vi "InitializeAnalogOutputforPADwithRamp.vi"(0 "AOTF":u16(ring) items=["None", "Laser 1", "Laser 2", "Laser 1 + 2", "Laser 3", "Laser 1 + 3", "Laser 2 + 3", "Laser 1+2+3", "Laser 1+2+3+4", "Laser 2+3+4"]) -> ()   [LabVIEW 2009]
uses:
  AnalogTrace.ctt
  TimingInfo.ctt
  <vilib>/Waveform/WDTOps.llb/WDT Append Waveforms DBL.vi
panel:
  in  "signal out":waveform(dbl)={"t0"=timestamp(0 s since 1904-01-01), "dt"=0.0, "Y"=[]}
  in  "Trace":T1
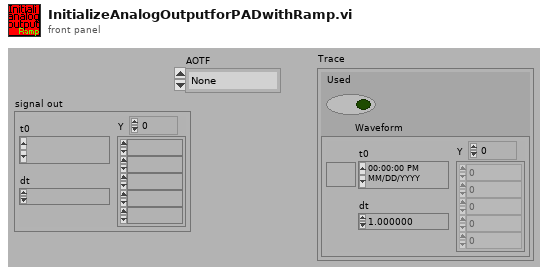
[diagram p1: front panel]
types:
  T1 = typedef "AnalogTrace.ctt" = cluster{"Used":bool, "Waveform":waveform(dbl)}
  T2 = cluster{"used":bool, "steps":u16, "start (V)":dbl, "stop (V)":dbl, "periode (s)":dbl, "manual":dbl[][]}
  T3 = typedef "TimingInfo.ctt" = cluster{"Fs":dbl, "#s":dbl}
  T4 = typedef "FIFOSettings.ctt" = cluster{"Measurement":cluster{"Binning (ms)":sgl, "External Trigger Condition":u16, "Stop Condition:":u16, "Stop Count":dbl, "Buffer Size (Photons)":u32, "No of Channels":u16, "Ext Latch Delay":i16}, "ADC":cluster{"Binning (HH)":i16, "Dither Range":i16, "Count Increment":i16, "Mode":u16}, "SYNC":cluster{"SYNC ZC Level (mV)":sgl, "SYNC Freq Divider":u16, "SYNC Holdoff (ps)":sgl, "SYNC Threshold (mV)":sgl}, "TAC":cluster{"TAC Range (ns)":sgl, "TAC Gain":i16, "TAC Offset (%)":sgl, "TAC Limit Low (%)":sgl, "TAC Limit High (%)":sgl}, "Ch 2":cluster{"Ch2 ZC Level (mV)":sgl, "Ch2 Holdoff (ps)":sgl, "Ch2 Threshold (mV)":sgl}, "Ch 3":cluster{"Ch3 ZC Level (mV)":sgl, "Ch3 Holdoff (ps)":sgl, "Ch3 Threshold (mV)":sgl}, "Ch 4":cluster{"Ch4 ZC Level (mV)":sgl, "Ch4 Holdoff (ps)":sgl, "Ch4 Threshold (mV)":sgl}, "Ch1":cluster{"Ch1 ZC Level (mV)":sgl, "Ch1 Holdoff (ps)":sgl, "Ch1 Threshold (mV)":sgl}}
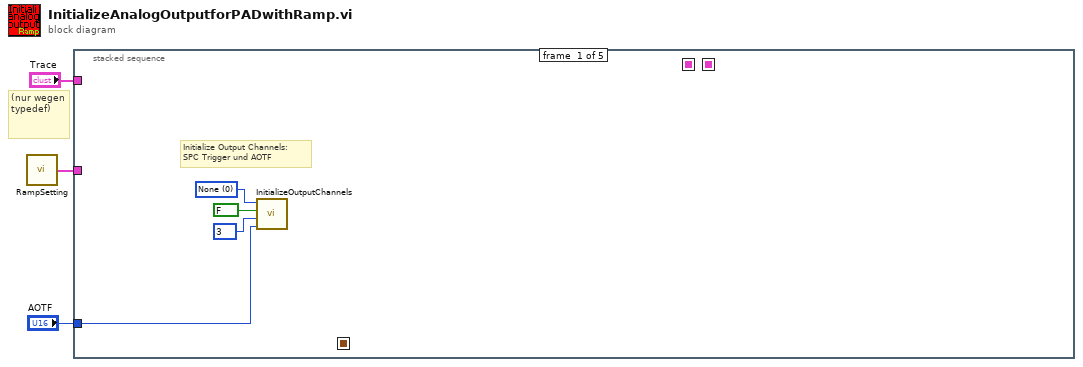
[diagram p0: block diagram]
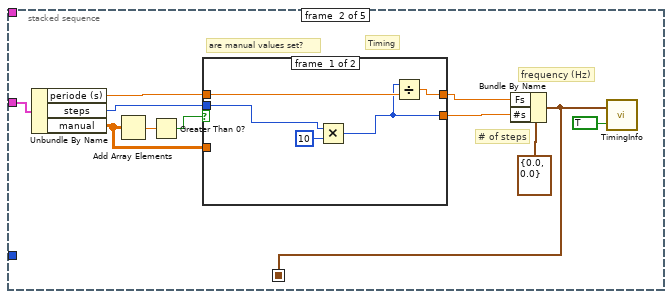
[diagram p2: hidden frame]
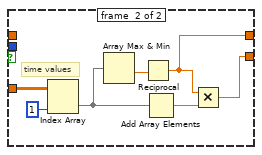
[diagram p3: hidden frame]
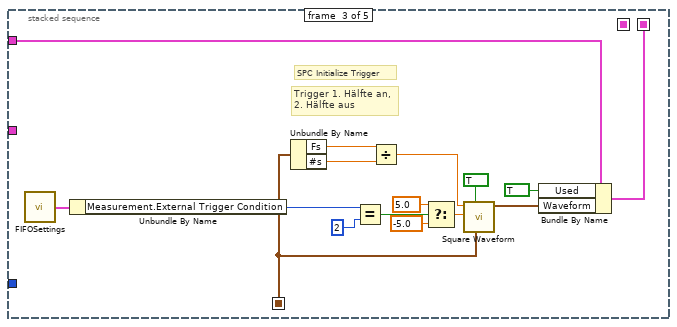
[diagram p4: hidden frame]
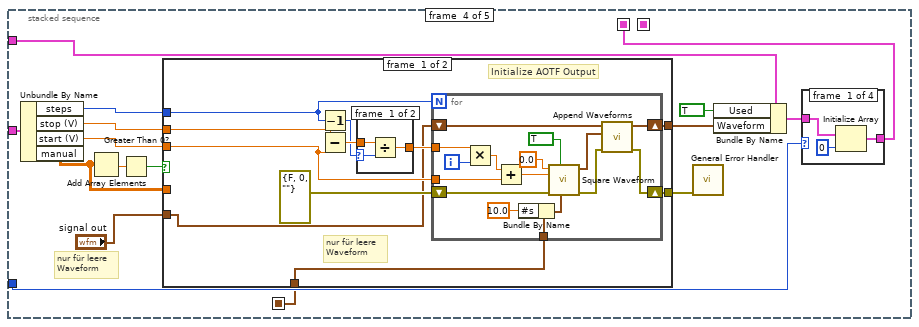
[diagram p5: hidden frame]
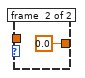
[diagram p6: hidden frame]
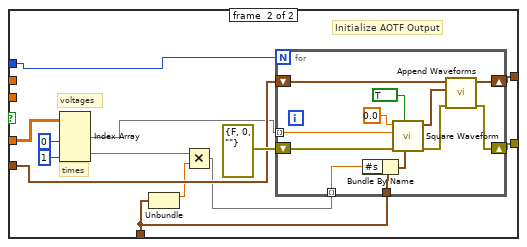
[diagram p7: hidden frame]
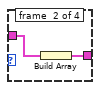
[diagram p8: hidden frame]
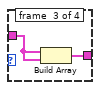
[diagram p9: hidden frame]
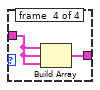
[diagram p10: hidden frame]
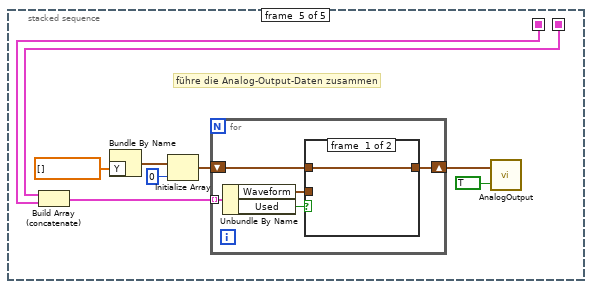
[diagram p11: hidden frame]
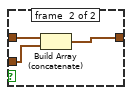
[diagram p12: hidden frame]
diagram:
  # "(nur wegen typedef)"
  n1 = call "RampSetting.vi"() -> ("RampSetting (out)"=w2:T2)  [unwired: 2 in]
  n2 = stacked-sequence {
    seq-local: [_ w15 _ _ _] -> [_ _ w35 w54 _]
    seq-local: [_ _ w34 _ _] -> [_ _ _ _ w129]
    seq-local: [_ _ _ w55 _] -> [_ _ _ _ w128]
    tunnel: "AOTF" -> [w4 _ _ w57 _]
    tunnel: w2 -> [_ w16 _ w56 _]
    tunnel: "Trace" -> [_ _ w33 w51 _]
    frame #0 {
      w7 = u16 0 items=["None", "Trace", "Retrace", "All"] ("EOM")
      w6 = u16 3 items=["x", "y", "z", ""] ("1st Axis")
      # "Initialize Output Channels:\nSPC Trigger und AOTF"
      n3 = call "InitializeOutputChannels.vi"("AOTF"=w4, "1st Axis"=w6, "Retrace"=FALSE, "EOM"=w7) -> ()
    }
    frame #1 {
      # "# of steps"
      # "frequency (Hz)"
      # "are manual values set?"
      # "Timing"
      n4 = Unbundle By Name(w16) -> ("periode (s)"=w13:dbl, "steps"=w12:u16, "manual"=w10:dbl[][])
      n5 = Add Array Elements(numeric array=w10) -> (sum=w14:dbl)
      n6 = Greater Than 0?(x=w14) -> (x > 0?=w11:bool)
      n7 = case shown="True" w11 {
        tunnel: [w19 w25] -> w8
        tunnel: w13 -> [w21 _]
        tunnel: [w20 w24] -> w9
        tunnel: w12 -> [w22 _]
        tunnel: w10 -> [_ w29]
        frame #0 {
          n8 = Multiply(x=w22, y=u16 10) -> (x*y=w20:u16)
          n9 = Divide(x=w20, y=w21) -> (x/y=w19:dbl)
        }
        frame #1 {
          # "time values"
          n10 = Index Array(array=w29, index (col)=1 ("disabled index (col)")) -> (element=w27:dbl[])  [unwired: 1 in]
          n11 = Array Max & Min(array=w27) -> (min value=w28:dbl)  [unwired: 3 out]
          n12 = Reciprocal(x=w28) -> (1/x=w25:dbl)
          n13 = Add Array Elements(numeric array=w27) -> (sum=w26:dbl)
          n14 = Multiply(x=w25, y=w26) -> (x*y=w24:dbl)
        }
      }
      n15 = Bundle By Name(cluster=T3 {"Fs"=0.0, "#s"=0.0} ("Timing Info"), "Fs"=w8, "#s"=w9) -> (w15:T3)
      n16 = call "TimingInfo.vi"("Get/Set"=TRUE, "Timing Info (input)"=w15) -> ()  [unwired: 1 out]
    }
    frame #2 {
      # "Trigger 1. Hälfte an, 2. Hälfte aus"
      # "SPC Initialize Trigger"
      n17 = call "FIFOSettings.vi"() -> ("FIFO Settings(out)"=w36:T4)  [unwired: 2 in]
      n18 = Unbundle By Name(w36) -> ("Measurement.External Trigger Condition"=w37:u16)
      n19 = Unbundle By Name(w35) -> ("Fs"=w46:dbl, "#s"=w32:dbl)
      n20 = Equal?(x=w37, y=u16 2) -> (x = y?=w41:bool)
      n21 = Divide(x=w46, y=w32) -> (x/y=w31:dbl)
      n22 = Select(t=5.0, s=w41, f=-5.0) -> (s? t:f=w45:dbl)
      n23 = call "Square Waveform.vi"("sampling info"=w35, "reset signal"=TRUE, "amplitude"=w45, "frequency"=w31) -> ("signal out"=w44:waveform(dbl))  [unwired: 6 in, 1 out]
      n24 = Bundle By Name(cluster=w33, "Used"=TRUE, "Waveform"=w44) -> (w34:T1)
    }
    frame #3 {
      # "nur für leere\nWaveform"
      n25 = Unbundle By Name(w56) -> ("steps"=w59:u16, "stop (V)"=w58:dbl, "start (V)"=w60:dbl, "manual"=w48:dbl[][])
      n26 = Add Array Elements(numeric array=w48) -> (sum=w50:dbl)
      n27 = Greater Than 0?(x=w50) -> (x > 0?=w49:bool)
      n28 = case shown="True" w49 {
        tunnel: w60 -> [w73 _]
        tunnel: w59 -> [w72 w105]
        tunnel: w58 -> [w69 _]
        tunnel: w54 -> [w68 w97]
        tunnel: [w67 w104] -> w53
        tunnel: [w66 w103] -> w52
        tunnel: w48 -> [_ w101]
        tunnel: "signal out" -> [w63 w102]
        frame #0 {
          # "nur für leere\nWaveform"
          # "Initialize AOTF Output"
          n29 = Decrement(x=w72) -> (x-1=w65:u16)
          n30 = Subtract(x=w69, y=w73) -> (x-y=w70:dbl)
          n31 = case shown="0" w65 {
            selector: w65 -> [w74 _]
            tunnel: [w76 0.0] -> w71
            tunnel: w70 -> [w75 _]
            frame #0 {
              n32 = Divide(x=w75, y=w74) -> (x/y=w76:dbl)
            }
            frame #1 {
            }
          }
          n33 = for {
            N: w72 -> [_]
            tunnel: w71 -> [w92]
            tunnel: w73 -> [w81]
            tunnel: w68 -> [w88]
            shift-right: [w85] -> w67
            shift-left: w63 -> [w84]
            shift-right: [w78] -> w66
            shift-left: errorcluster {"status"=FALSE, "code"=0, "source"=""} ("error out") -> [w79]
            i -> [w93]
            n34 = Multiply(x=w92, y=w93) -> (x*y=w82:dbl)
            n35 = Add(x=w82, y=w81) -> (x+y=w90:dbl)
            n36 = Bundle By Name(cluster=w88, "#s"=10.0) -> (w87:T3)
            n37 = call "Square Waveform.vi"("sampling info"=w87, "reset signal"=TRUE, "error in (no error)"=w79, "amplitude"=w90, "frequency"=0.0) -> ("error out"=w80:errorcluster, "signal out"=w89:waveform(dbl))  [unwired: 5 in]
            n38 = call-poly <vilib>:"Append Waveforms.vi"("error in (no error)"=w80, "waveform B"=w89, "waveform A"=w84) -> ("error out"=w78:errorcluster, "waveform out"=w85:waveform(dbl))  [unwired: 7 in]
          }
        }
        frame #1 {
          # "times"
          # "voltages"
          # "Initialize AOTF Output"
          n39 = Index Array(array=w101, index (col) #1=0 ("disabled index (col)"), index (col) #2=1 ("index (col)")) -> (element #1=w99:dbl[], element #2=w96:dbl[])  [unwired: 2 in]
          n40 = Unbundle(w97) -> ("Fs"=w94:dbl)  [unwired: 1 out]
          n41 = Multiply(x=w96, y=w94) -> (x*y=w95:dbl[])
          n42 = for {
            N: w105 -> [_]
            tunnel: w97 -> [w116]
            shift-right: [w114] -> w104
            shift-left: w102 -> [w113]
            shift-right: [w109] -> w103
            shift-left: errorcluster {"status"=FALSE, "code"=0, "source"=""} ("error out") -> [w110]
            tunnel: w99 -> [w108] mode=indexing
            tunnel: w95 -> [w107] mode=indexing
            n43 = Bundle By Name(cluster=w116, "#s"=w107) -> (w115:T3)
            n44 = call "Square Waveform.vi"("sampling info"=w115, "reset signal"=TRUE, "error in (no error)"=w110, "amplitude"=w108, "frequency"=0.0) -> ("error out"=w111:errorcluster, "signal out"=w117:waveform(dbl))  [unwired: 5 in]
            n45 = call-poly <vilib>:"Append Waveforms.vi"("error in (no error)"=w111, "waveform B"=w117, "waveform A"=w113) -> ("error out"=w109:errorcluster, "waveform out"=w114:waveform(dbl))  [unwired: 7 in]
          }
        }
      }
      n46 = call <vilib>:"General Error Handler.vi"("error in (no error)"=w52) -> ()  [unwired: 10 in, 5 out]
      n47 = Bundle By Name(cluster=w51, "Used"=TRUE, "Waveform"=w53) -> (w62:T1)
      n48 = case shown="0, Default" w57 {
        tunnel: w62 -> [w120 w123 w125 w127]
        tunnel: [w121 w122 w124 w126] -> w55
        frame #0 {
          n49 = Initialize Array(w120, 0 ("dimension size")) -> (w121:T1[])
        }
        frame #1 {
          n50 = Build Array(w123) -> (w122:T1[])
        }
        frame #2 {
          n51 = Build Array(w125, w125) -> (w124:T1[])
        }
        frame #3 {
          n52 = Build Array(w127, w127, w127) -> (w126:T1[])
        }
      }
    }
    frame #4 {
      # "führe die Analog-Output-Daten zusammen"
      n53 = Build Array (concatenate)(w129, w128) -> (w136:T1[])
      n54 = Bundle By Name("Y"=dbl[] []) -> (w133:waveform(dbl))  [unwired: 1 in]
      n55 = Initialize Array(w133, 0 ("dimension size")) -> (w134:waveform(dbl)[])
      n56 = for {
        shift-right: [w139] -> w135
        shift-left: w134 -> [w138]
        tunnel: w136 -> [w141] mode=indexing
        n57 = Unbundle By Name(w141) -> ("Waveform"=w137:waveform(dbl), "Used"=w140:bool)
        n58 = case shown="True" w140 {
          tunnel: [w142 w145] -> w139
          tunnel: w138 -> [w142 w144]
          tunnel: w137 -> [_ w143]
          frame #0 {
          }
          frame #1 {
            n59 = Build Array (concatenate)(w144, w143) -> (w145:waveform(dbl)[])
          }
        }
      }
      n60 = call "AnalogOutput.vi"("Get/Set"=TRUE, "Analog Output (input)"=w135) -> ()  [unwired: 1 out]
    }
  }
